vi "Direttore.rtloop.fpga.vi"() -> ()   [LabVIEW 2011]
uses:
  <vilib>/Platform/TimedLoop/XDataNode/timing_clust.ctl
  <vilib>/Platform/TimedLoop/XDataNode/nitl_modes.ctl
  <vilib>/Platform/TimedLoop/XDataNode/wakeup.ctl
  <vilib>/rvi/Memory/Memory_Emulation/niFpgaMemoryEmulationValidateCache.vi
  <vilib>/rvi/DataTransferAndStorage/Container/Common/niFpgaContainerGetUniqueNameForEmu.vi
  <vilib>/rvi/Memory/Memory_Emulation/nirvimemoryEmulationManagerCache_InsertValue.vi
  <vilib>/Utility/error.llb/Clear Errors.vi
  <vilib>/rvi/Memory/Memory_Emulation/nirvimemoryEmulationManagerCache_GetValue.vi
  <vilib>/rvi/Memory/Memory_Emulation/nirvimemoryEmulationManagerCache_SetValue.vi
  <vilib>/Platform/TimedLoop/XDataNode/XDataNode.xnode
  <vilib>/rvi/DataTransferAndStorage/Container/XNode/niFpgaContainer.xnode
  <vilib>/rvi/Memory/Memory_Emulation/nirvimemoryEmulation.vi
  <vilib>/Platform/TimedLoop/XDataNode/XDNodeRunTimeDep.lvlib
panel:
  out "Error":errorcluster
  out "InputMatrixElement":i16
  in  "GetInputmatrix":bool
  in  "OutputMatrixElement":i16
  in  "Address":u32
  in  "SetOutputMatrix":bool
  in  "PlayMatrix":bool
  in  "dt (uSec)":u32 caption="AI Count(uSec)"
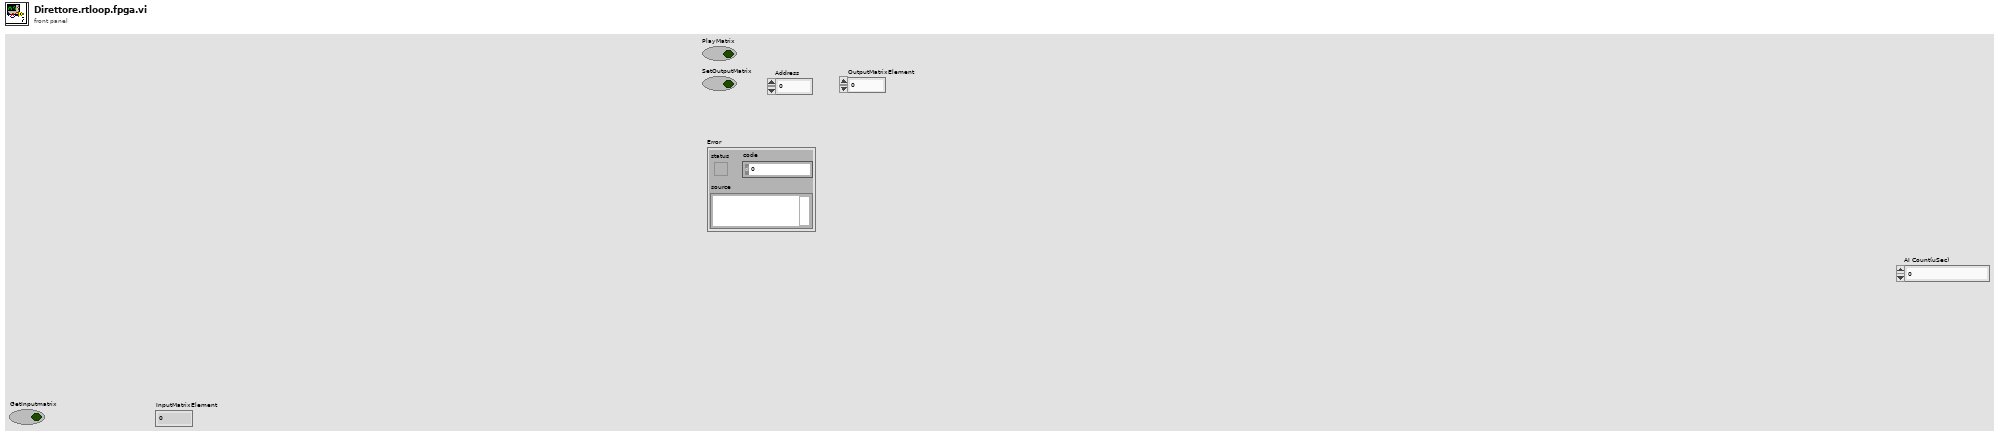
[diagram p1: front panel]
types:
  T1 = typedef "XDNodeRunTimeDep.lvlib/timing_clust.ctl" = cluster{"Expected End [f-1]":u64, "Actual End [f-1]":u64, "Finished Late? [f-1]":bool, "Expected End [i-1]":u64, "Actual End [i-1]":u64, "Finished Late? [i-1]":bool, "Expected Start [i]":u64, "Actual Start [i]":u64, "Expected Start [f]":u64, "Actual Start [f]":u64, "Source Name":string, "Structure Name":string, "Period":i64, "Deadline":i64, "Offset":i64, "Start":i64, "Priority":i32, "Timeout":i32, "Mode":T2, "Wakeup Reason":T3, "Error":errorcluster, "Source Type":string, "Secondary Source Type":string, "Global End Time":u64, "Global Start Time":u64, "Frame Duration":u64, "Iteration Duration":u64, "Assigned CPU":i32, "I/O Scan Engine Mode":u32}
  T2 = typedef "XDNodeRunTimeDep.lvlib/nitl_modes.ctl" = enum32{"No Change", "Process missed periods, maintain original phase", "Discard missed periods, maintain original phase", "Process missed periods, ignore original phase", "Discard missed periods, ignore original phase"}
  T3 = typedef "XDNodeRunTimeDep.lvlib/wakeup.ctl" = enum32{"Normal", "Aborted", "Asynchronous wakeup", "Timing source error", "Timed loop error", "Timeout"}
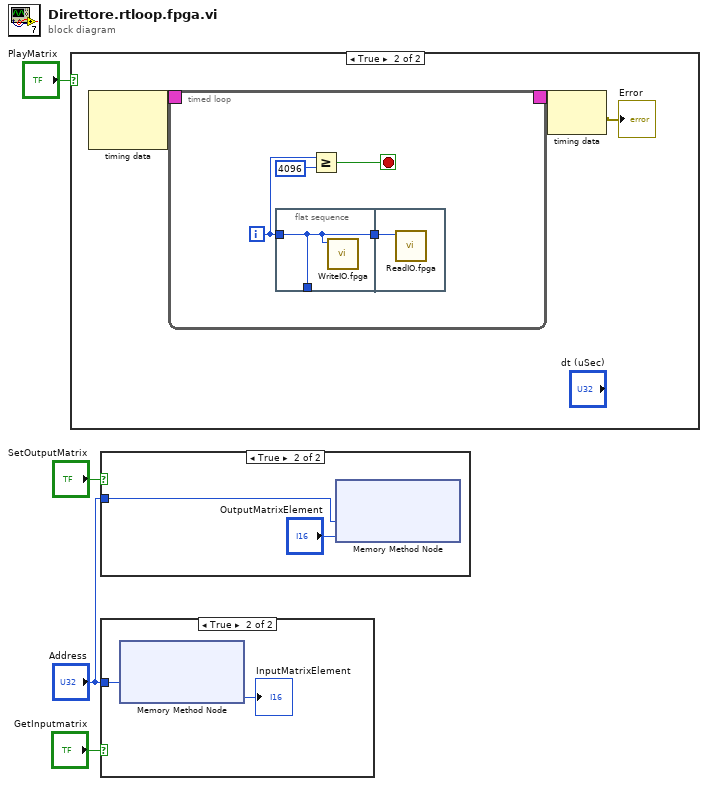
[diagram p0: block diagram]
diagram:
  n1 = case shown="True" "PlayMatrix" {
    frame False {
    }
    frame True {
      n2 = node-c288() -> (w7:T1)  [unwired: 2 in]
      n3 = timed-loop {
        timing: w7 -> [_]
        timing-out: [_] -> w6
        i -> [w8]
        stop <- w10 stop-if-true
        n4 = flat-sequence {
          tunnel: [w12] -> _
          tunnel: [w12] -> w11
          tunnel: w8 -> [w12]
          tunnel: w11 -> [w13]
          frame #0 {
            n5 = call "WriteIO.fpga.vi"("x"=w12) -> ()  [unwired: 11 in]
          }
          frame #1 {
            n6 = call "ReadIO.fpga.vi"("x"=w13) -> ()  [unwired: 11 in]
          }
        }
        n7 = Greater Or Equal?(x=w8, y=u32 4096) -> (x >= y?=w10:bool)
      }
      n8 = node-c288(w6) -> (→"Error":errorcluster)
    }
  }
  n9 = case shown="True" "SetOutputMatrix" {
    tunnel: "Address" -> [_ w19]
    frame False {
    }
    frame True {
      n10 = xnode ("Memory Method Node")("Address"=w19, "Data"="OutputMatrixElement") -> ()  [unwired: 1 in, 1 out]
    }
  }
  n11 = case shown="True" "GetInputmatrix" {
    tunnel: "Address" -> [_ w21]
    frame False {
    }
    frame True {
      n12 = xnode ("Memory Method Node")("Address"=w21) -> ("Data"=→"InputMatrixElement":i16)  [unwired: 1 in, 1 out]
    }
  }
